vi "Subscribe.vi"(7 "Enqueuer ID string":string, 8 "error in (no error)":errorcluster, 9 "Data Array":refnum<class "Data.lvclass">[](array[class]), 10 "Message Array":refnum<class "Message.lvclass">[](array[class]), 11 "Publisher in":refnum<class "Publisher.lvclass">) -> (0 "error out":errorcluster, 1 "Success?":bool, 3 "Publisher out":refnum<class "Publisher.lvclass">)   [LabVIEW 2020, in "Publisher.lvlib" / "Publisher.lvclass"]
doc: "Setup up a subscription for the actor with 'Enqueuer ID'."
uses:
  Publisher.lvclass
  PPL/HDH.Data.Generic.lvlibp/Data.lvclass
  PPL/HDH.Actor Framework.Core.Actor.lvlibp/1abvi3w/vi.lib/ActorFramework/Message/Message.lvclass
  Publisher.lvclass/Publisher.ctl
  PPL/HDH.Actor Framework.Core.Actor.lvlibp/1abvi3w/vi.lib/ActorFramework/Message Enqueuer/Message Enqueuer.lvclass
  Add Subscriber.vi/9bfa7042-f496-41a0-bdb3-f05adf9a1a12.vi
  PPL/HDH.Actor Framework.Core.Utility.lvlibp/Object/To Default Object.vi
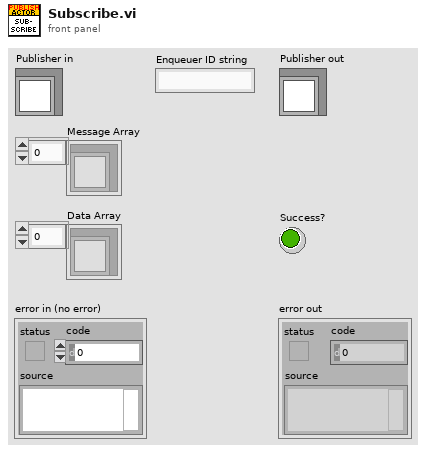
[diagram p1: front panel]
types:
  T1 = typedef "Publisher.lvlib/Publisher.lvclass/Ctl_Subscription Element.ctl" = cluster{"Object":refnum<class>, "Enqueuers":refnum<class "Message Enqueuer.lvclass">[]}
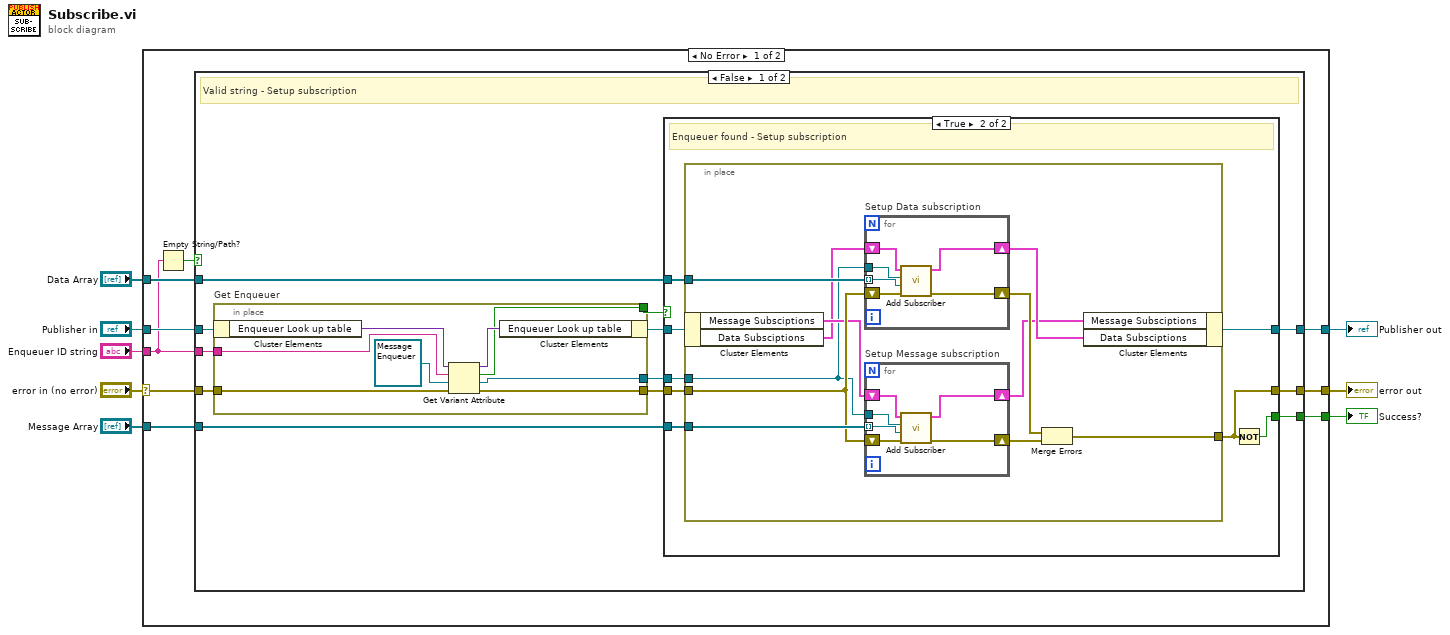
[diagram p0: block diagram]
diagram:
  n1 = case shown="No Error" "error in (no error)" {
    selector: "error in (no error)" -> [w14 w75]
    tunnel: [w13 w75] -> w7
    tunnel: [w16 w74] -> w5
    tunnel: "Publisher in" -> [w17 w74]
    tunnel: "Message Array" -> [w9 _]
    tunnel: "Data Array" -> [w15 _]
    tunnel: "Enqueuer ID string" -> [w11 _]
    tunnel: [w12 _] -> w1
    frame No Error {
      n2 = Empty String/Path?(string/path=w11) -> (empty?=w10:bool)
      n3 = case shown="False" w10 {
        tunnel: w11 -> [w29 _]
        tunnel: w17 -> [w26 w73]
        tunnel: [w24 w73] -> w16
        tunnel: w15 -> [w23 _]
        tunnel: w14 -> [w22 w72]
        tunnel: [w21 w72] -> w13
        tunnel: [w19 _] -> w12
        tunnel: w9 -> [w18 _]
        frame False {
          # "Valid string - Setup subscription"
          n4 = in-place "Get Enqueuer" {
            in-place-border: w29 -> [w70]
            in-place-border: [w67] -> w28
            in-place-border: [w66] -> w27
            in-place-border: w22 -> [w65]
            in-place-border: [w64] -> w20
            n5 = in-place-cluster #1(w26) -> ("Enqueuer Look up table"=w71:variant)
            n6 = Get Variant Attribute(Variant=w71, name=w70, default value (empty Variant)=refnum<class "Message Enqueuer.lvclass"> refnum ("Message Enqueuer in"), error in=w65) -> (duplicate Variant=w68:variant, found=w67:bool, value=w66:refnum<class "Message Enqueuer.lvclass">, error out=w64:errorcluster)
            n7 = in-place-cluster #1("Enqueuer Look up table"=w68) -> (w25:refnum<class "Publisher.lvclass">)
          }
          n8 = case shown="True" w28 {
            selector: w28 -> [w30 _]
            tunnel: w27 -> [_ w36]
            tunnel: [w32 w33] -> w24
            tunnel: w25 -> [w32 w40]
            tunnel: w23 -> [_ w37]
            tunnel: [w31 w35] -> w21
            tunnel: w20 -> [w31 w38]
            tunnel: [w30 w34] -> w19
            tunnel: w18 -> [_ w39]
            frame False {
              # "Enqueuer not found - No success"
            }
            frame True {
              # "Enqueuer found - Setup subscription"
              n9 = in-place {
                in-place-border: w39 -> [w51]
                in-place-border: w38 -> [w49]
                in-place-border: [w47] -> w35
                in-place-border: w37 -> [w48]
                in-place-border: w36 -> [w41]
                n10 = in-place-cluster #2(w40) -> ("Message Subsciptions"=w45:T1[], "Data Subsciptions"=w44:T1[])
                n11 = for "Setup Data subscription" {
                  tunnel: w48 -> [w59] mode=indexing
                  shift-right: [w61] -> w46
                  shift-left: w49 -> [w58]
                  shift-right: [w62] -> w43
                  shift-left: w44 -> [w63]
                  tunnel: w41 -> [w60]
                  n12 = call "Add Subscriber.vi"("error in (no error)"=w58, "Subscription Object"=w59, "Subscriber Enqueuer"=w60, "Subsciptions in"=w63) -> ("error out"=w61:errorcluster, "Subsciptions out"=w62:T1[])  [unwired: 6 in]
                }
                n13 = for "Setup Message subscription" {
                  tunnel: w51 -> [w52] mode=indexing
                  shift-right: [w56] -> w50
                  shift-left: w49 -> [w53]
                  shift-right: [w57] -> w42
                  shift-left: w45 -> [w55]
                  tunnel: w41 -> [w54]
                  n14 = call "Add Subscriber.vi"("error in (no error)"=w53, "Subscription Object"=w52, "Subscriber Enqueuer"=w54, "Subsciptions in"=w55) -> ("error out"=w56:errorcluster, "Subsciptions out"=w57:T1[])  [unwired: 6 in]
                }
                n15 = Merge Errors(w46, w50) -> (w47:errorcluster)
                n16 = in-place-cluster #2("Message Subsciptions"=w42, "Data Subsciptions"=w43) -> (w33:refnum<class "Publisher.lvclass">)
              }
              n17 = Not(x=w35) -> (.not. x?=w34:bool)
            }
          }
        }
        frame True {
          # "Invalid string - No success"
        }
      }
    }
    frame Error {
    }
  }
  "error out" <- w7
  "Publisher out" <- w5
  "Success?" <- w1
